vi "Excel表格写.vi"(8 "表格":string[][](table), 9 "单页表名称":string="接触面", 10 "列首":string[](array[string]) caption="行首", 11 "路径":path=path "E:/广东华旃/广东华旃864插座位置度CCD检测-all/广东华旃插座位置度CCD检测-20200721/接触面PIN 正位度-864 设备调试比对-3号样品-7.16.xlsx") -> (1 "写表格结果":bool)   [LabVIEW 2014]
uses:
  <vilib>/Utility/file.llb/Write To Spreadsheet File (string).vi
  <vilib>/Utility/NIReport.llb/NI_report.lvclass
  <vilib>/Utility/NIReport.llb/Excel/NI_Excel.lvclass
  <vilib>/Utility/NIReport.llb/Append Text Table to Report (wrap).vi
panel:
  in  "路径 2":path=path "E:/广东华旃/广东华旃864插座位置度CCD检测-all/广东华旃插座位置度CCD检测-20200721/接触面PIN 正位度-864 设备调试比对-3号样品-7.16.xlsx"
  out "输出数组":string[][](array[string])
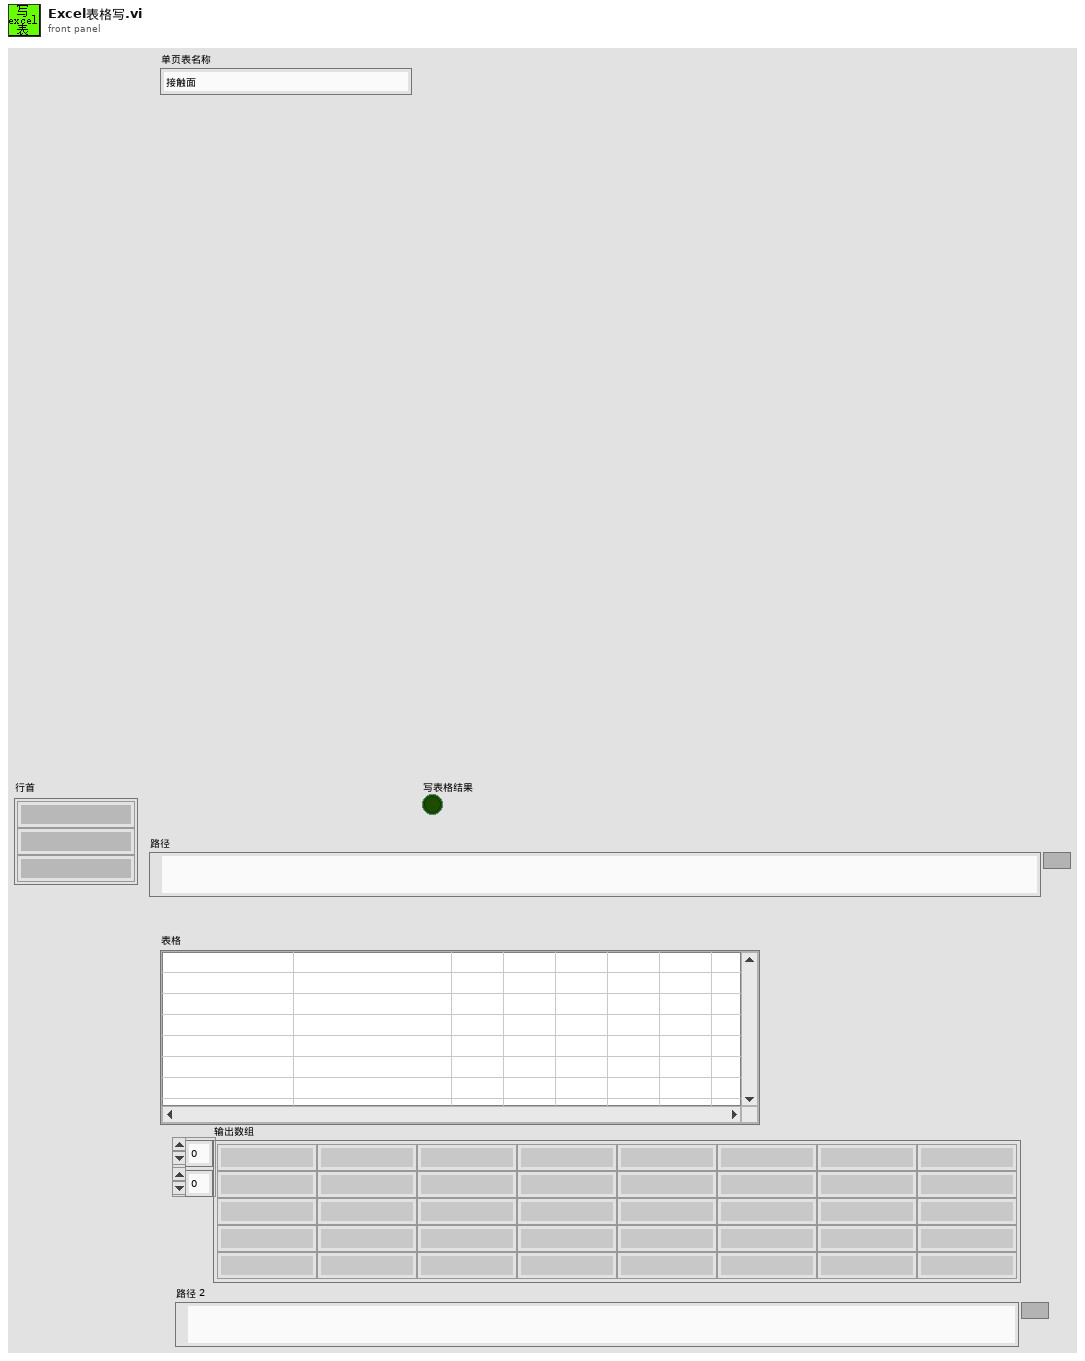
[diagram p1: front panel]
types:
  T1 = cluster{"position (excel)":cluster{"row":i32, "column":i32}, "name (excel)":string, "bookmark (word)":string}
  T2 = enum16{"maximized", "minimized", "normal", "no change"}
  T3 = enum16{"Standard Report", "HTML", "Word", "Excel"}
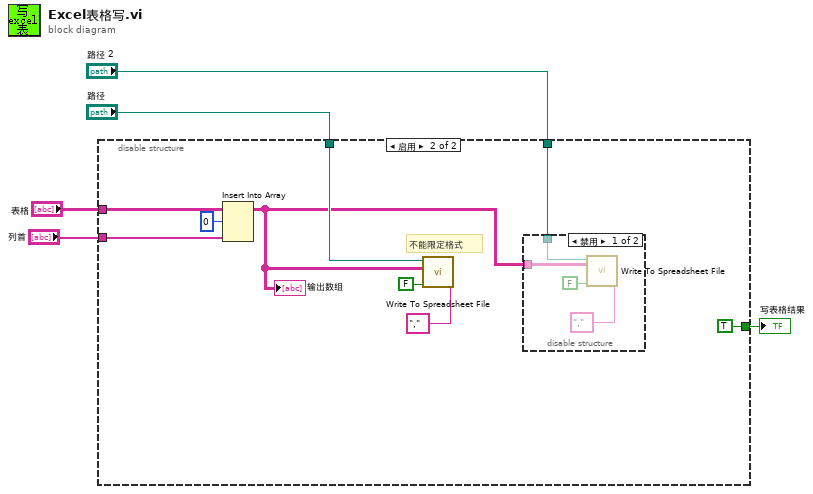
[diagram p0: block diagram]
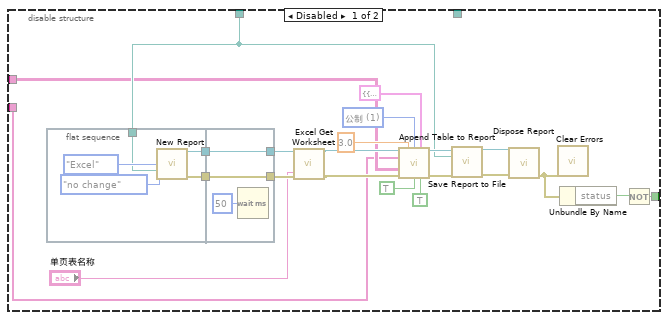
[diagram p2: hidden frame]
diagram:
  n1 = disable-structure shown="启用" {
    disable-tunnel: [w11 TRUE ("写表格结果")] -> w5
    disable-tunnel: "路径" -> [w10 w39]
    disable-tunnel: "表格" -> [w7 w42]
    disable-tunnel: "列首" -> [w6 w41]
    disable-tunnel: "路径 2" -> [_ w37]
    frame Disabled {
      w22 = u16 1 items=["US", "公制", "默认"] ("measurement system")
      n2 = flat-sequence {
        tunnel: [w32] -> w27
        tunnel: w10 -> [w29]
        tunnel: [w28] -> w26
        tunnel: [w35] -> w25
        tunnel: w27 -> [w35]
        tunnel: [w33] -> w24
        tunnel: w26 -> [w33]
        frame #0 {
          n3 = call <vilib>:"New Report.vi"("window state (normal)"=T2."no change", "report type"=T3."Excel", "template (empty)"=w29) -> ("report out"=w32:refnum<class "NI_report.lvclass">, "error out"=w28:errorcluster)  [unwired: 11 in]
        }
        frame #1 {
          n4 = Wait (ms)(milliseconds to wait=u32 50 ("等待时间（毫秒）")) -> ()  [unwired: 1 out]
        }
      }
      n5 = call <vilib>:"Excel Get Worksheet.vi"("report in"=w25, "error in (no error)"=w24, "name (\"\")"="单页表名称") -> ("report out"=w17:refnum<class "NI_report.lvclass">, "error out"=w16:errorcluster)  [unwired: 11 in]
      n6 = call-poly <vilib>:"Append Table to Report.vi"("report in"=w17, "column width (1)"=3.0, "measurement system"=w22, "MS Office parameters"=T1 {"position (excel)"={"row"=0, "column"=0}, "name (excel)"="", "bookmark (word)"=""}, "column headers"=w6, "text data"=w7, "error in (no error)"=w16, "separate page? (NO)"=TRUE, "show grid lines (YES)"=TRUE) -> ("report out"=w18:refnum<class "NI_report.lvclass">, "error out"=w19:errorcluster)  [unwired: 3 in, 2 out]
      n7 = call-dynamic "Save Report to File.vi"("report in"=w18, "report file path"=w10, "error in (no error)"=w19) -> ("report out"=w14:refnum<class "NI_report.lvclass">, "error out"=w15:errorcluster)  [unwired: 11 in]
      n8 = call-dynamic "Dispose Report.vi"("report in"=w14, "error in (no error)"=w15) -> ("error out"=w13:errorcluster)  [unwired: 13 in]
      n9 = call <vilib>:"Clear Errors.vi"("error in (no error)"=w13) -> ()  [unwired: 5 in, 2 out]
      n10 = Unbundle By Name(w13) -> ("status"=w12:bool)
      n11 = Not(x=w12) -> (.not. x?=w11:bool)
    }
    frame Enabled {
      # "不能限定格式"
      n12 = Insert Into Array(array=w42, index (row)=0 ("索引 (行)"), new element=w41) -> (w38:string[][])  [unwired: 1 in]
      "输出数组" <- w38
      n13 = call-poly <vilib>:"Write To Spreadsheet File.vi"("delimiter (\\t)"="," ("delimiter (\\t)"), "append to file? (new file:F)"=FALSE, "2D data"=w38, "file path (dialog if empty)"=w39) -> ()  [unwired: 4 in, 1 out]
      n14 = disable-structure shown="禁用" {
        disable-tunnel: w38 -> [w47 _]
        disable-tunnel: w37 -> [w45 _]
        frame Disabled {
          n15 = call-poly <vilib>:"Write To Spreadsheet File.vi"("delimiter (\\t)"="," ("delimiter (\\t)"), "append to file? (new file:F)"=FALSE, "2D data"=w47, "file path (dialog if empty)"=w45) -> ()  [unwired: 4 in, 1 out]
        }
        frame Enabled {
        }
      }
    }
  }
  "写表格结果" <- w5
